vi "Test.vi"() -> ()   [LabVIEW 2017]
uses:
  <instrlib>/Mercury iXX/Public/Controls/Comms Transport Layer.ctl
  <instrlib>/Mercury iXX/Public/Controls/Unit String.ctl
  <instrlib>/Mercury iXX/Public/Libraries/System/Open/Open System.vi
  <instrlib>/Mercury iXX/Public/Libraries/System/Read/Catalogue (Read).vi
  <instrlib>/Mercury iXX/Public/Libraries/Temperature/Open/Open Temperature Device.vi
  <instrlib>/Mercury iXX/Public/Libraries/Temperature/Signals/Read/Temperature (Read).vi
  <vilib>/Utility/file.llb/Write Delimited Spreadsheet (string).vi
  ProgramData/Documents/Princeton Instruments/LightField/Add-in and Automation SDK/Samples/LabVIEW Automation/lightfield-automation-labview/LightField Automation.lvclass
  <instrlib>/Mercury iXX/Mercury iXX.lvlib
  <instrlib>/Quantum Composers 9000 Series 2.08/Quantum Composers 9000 Series.lvlib
  <instrlib>/Mercury iXX/Public/Libraries/Temperature.lvlib
  <instrlib>/Mercury iXX/Public/Libraries/System.lvlib
  <instrlib>/Tektronix TDS 200 1000 2000 Series/Tektronix TDS 200 1000 2000 Series.lvlib
  <instrlib>/Tektronix TDS 200 1000 2000 Series/Public/Data/Read (Multiple Waveforms).vi
  <vilib>/Waveform/WDTFileIO.llb/ Write Waveforms to File (1D).vi
  <vilib>/Waveform/WDTFileIO.llb/Export Waveforms To Spreadsheet File (1D).vi
  <instrlib>/Tektronix TDS 200 1000 2000 Series/Public/Configure/Configure Trigger (Edge).vi
panel:
  out "Array":string[](array[string])
  out "Array 2":string[](array[string])
  in  "?":bool
  in  "Turbulence Experiment":T1(tab)
  in  "VISA resource name":refnum<visa-resource-name>
  in  "Comms Layer":T2
  in  "Device Identifier":string="MB1.T1:TEMP"
  out "error out":errorcluster
  in  "Read Interval (s)":sgl=1.0 min=0.25 max=1000 step=0.25 format="%.2f"
  in  "Record Temperature Data":bool
  out "Unit":T3
  out "Temperature":dbl
  in  "Experiment Name":string="Experiment1"
  in  "Repetitive Gate Width (us)":dbl
  in  "Intensifier Gain":i32
  in  "Start":bool
  in  "?":bool
  in  "Time between frames":i32=500
  in  "On Chip Accumulations 2":i32=6
  in  "Number of Frames 2":i32
  in  "COM Port Settings":T4={"Unit ID"="A", "Baud Rate"=enum."19200", "VISA Sesssion In"="COM1"}
  out "Measurement Data":T5
  in  "Minimum time between \nreadings [ms]":u32
  out "Elapsed Time [ms]":dbl caption="Elapsed Time (s)"
  out "Measurements\nper second":dbl
  in  "End Program":bool
  out "Error Text":string
  out "Error Present":bool
  out "Range Exceeded":bool
  in  "Data Logging Options (If valid)":T6={"Absolute Press."=TRUE, "Gauge/Diff. Press."=TRUE, "Barometric Press."=TRUE, "Temperature"=TRUE, "Volumetric"=TRUE, "Mass Flow"=TRUE, "Setpoint"=TRUE, "Valve Drive"=FALSE, "Totalizer"=TRUE, "Tot. Timer [s]"=FALSE, "Tot. Avg. Flow"=FALSE, "Tot. Peak Flow"=FALSE, "Gas Selected"=TRUE, "Log Data"=TRUE}
  out "Commands":string
  in  "OK Button":bool
  in  "Command to Send":string
  out "Response from Alicat":string
  in  "End Program 2":bool
  in  "Data folder":path=path "C:/Data"
  in  "Oscilloscope":refnum<visa-resource-name>="USB0::0x0699::0x03A6::C016710::INSTR"
  in  "Pulse generater":refnum<visa-resource-name>="COM3"
  # "Stop Oscilloscope"
  # "Stop Lightfield"
  # "Totalizer Timer"
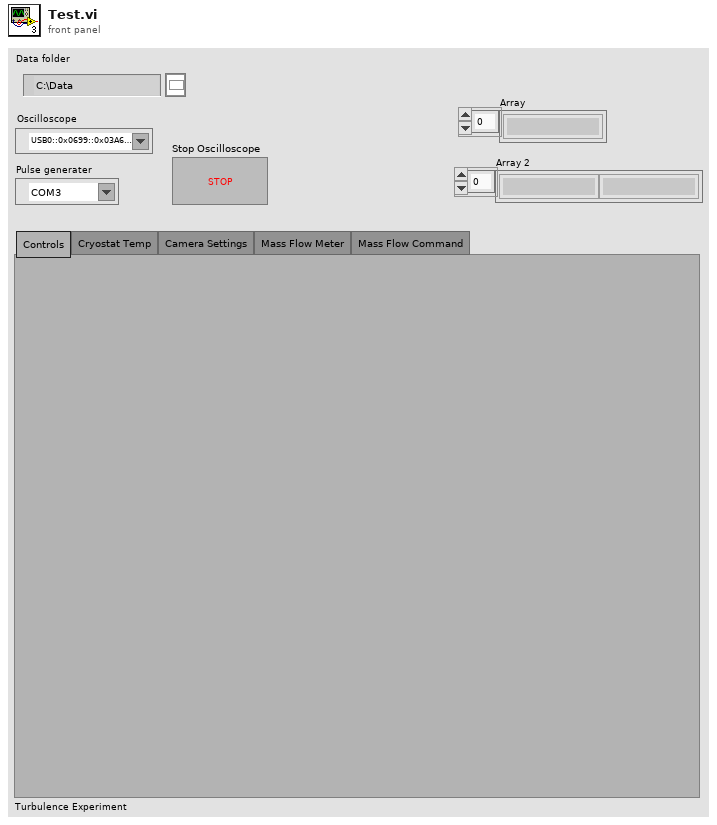
[diagram p1: front panel]
types:
  T1 = enum32{"Controls", "Cryostat Temp", "Camera Settings", "Mass Flow Meter", "Mass Flow Command"}
  T2 = typedef "Mercury iXX.lvlib/Comms Transport Layer.ctl" = enum16{"Ethernet TCP/IP", "USB", "ISOBus - RS-232", "GPIB"}
  T3 = typedef "Mercury iXX.lvlib/Unit String.ctl" = string
  T4 = cluster{"Unit ID":string, "Baud Rate":enum8{"2400", "9600", "19200", "38400", "57600", "115200", "Unknown"}, "VISA Sesssion In":refnum<visa-resource-name>}
  T5 = cluster{"Absolute Pressure":dbl, "Gauge/Diff. Pressure":dbl, "Barometric Pressure":dbl, "Temperature":dbl, "Volumetric Flow":dbl, "Mass Flow":dbl, "Setpoint":dbl, "Valve Drive":dbl, "Totalizer":dbl, "[hr]":dbl, "[min]":dbl, "[sec]":dbl, "Totalizer Average Flow":dbl, "Totalizer Peak Flow":dbl, "Gas selected":string}
  T6 = cluster{"Absolute Press.":bool, "Gauge/Diff. Press.":bool, "Barometric Press.":bool, "Temperature":bool, "Volumetric":bool, "Mass Flow":bool, "Setpoint":bool, "Valve Drive":bool, "Totalizer":bool, "Tot. Timer [s]":bool, "Tot. Avg. Flow":bool, "Tot. Peak Flow":bool, "Gas Selected":bool, "Log Data":bool}
  T7 = typedef "Mercury iXX.lvlib/Mercury Reference.ctl" = cluster{"Comms":refnum<visa-resource-name>, "Device ID":string[], "Comms Layer":T2, "Command":string, "Query reference":T8}
  T8 = typedef "Mercury iXX.lvlib/Query Dynamic Reference.ctl" = refnum<vi>
  T9 = enum16{"open", "replace", "create", "open or create", "replace or create", "replace or create with confirmation"}
  T10 = cluster{"Absolute Pressure":bool, "Gauge/Diff. Pressure":bool, "Barometric Pressure":bool, "Temperature":bool, "Volumetric":bool, "Mass":bool, "Setpoint":bool, "Valve Drive":bool, "Totalizer":bool, "Totalizer Timer":bool, "Totalizer Average Flow":bool, "Totalizer Peak Flow":bool, "Gas Selected":bool, "Tot. Timer Format":u16}
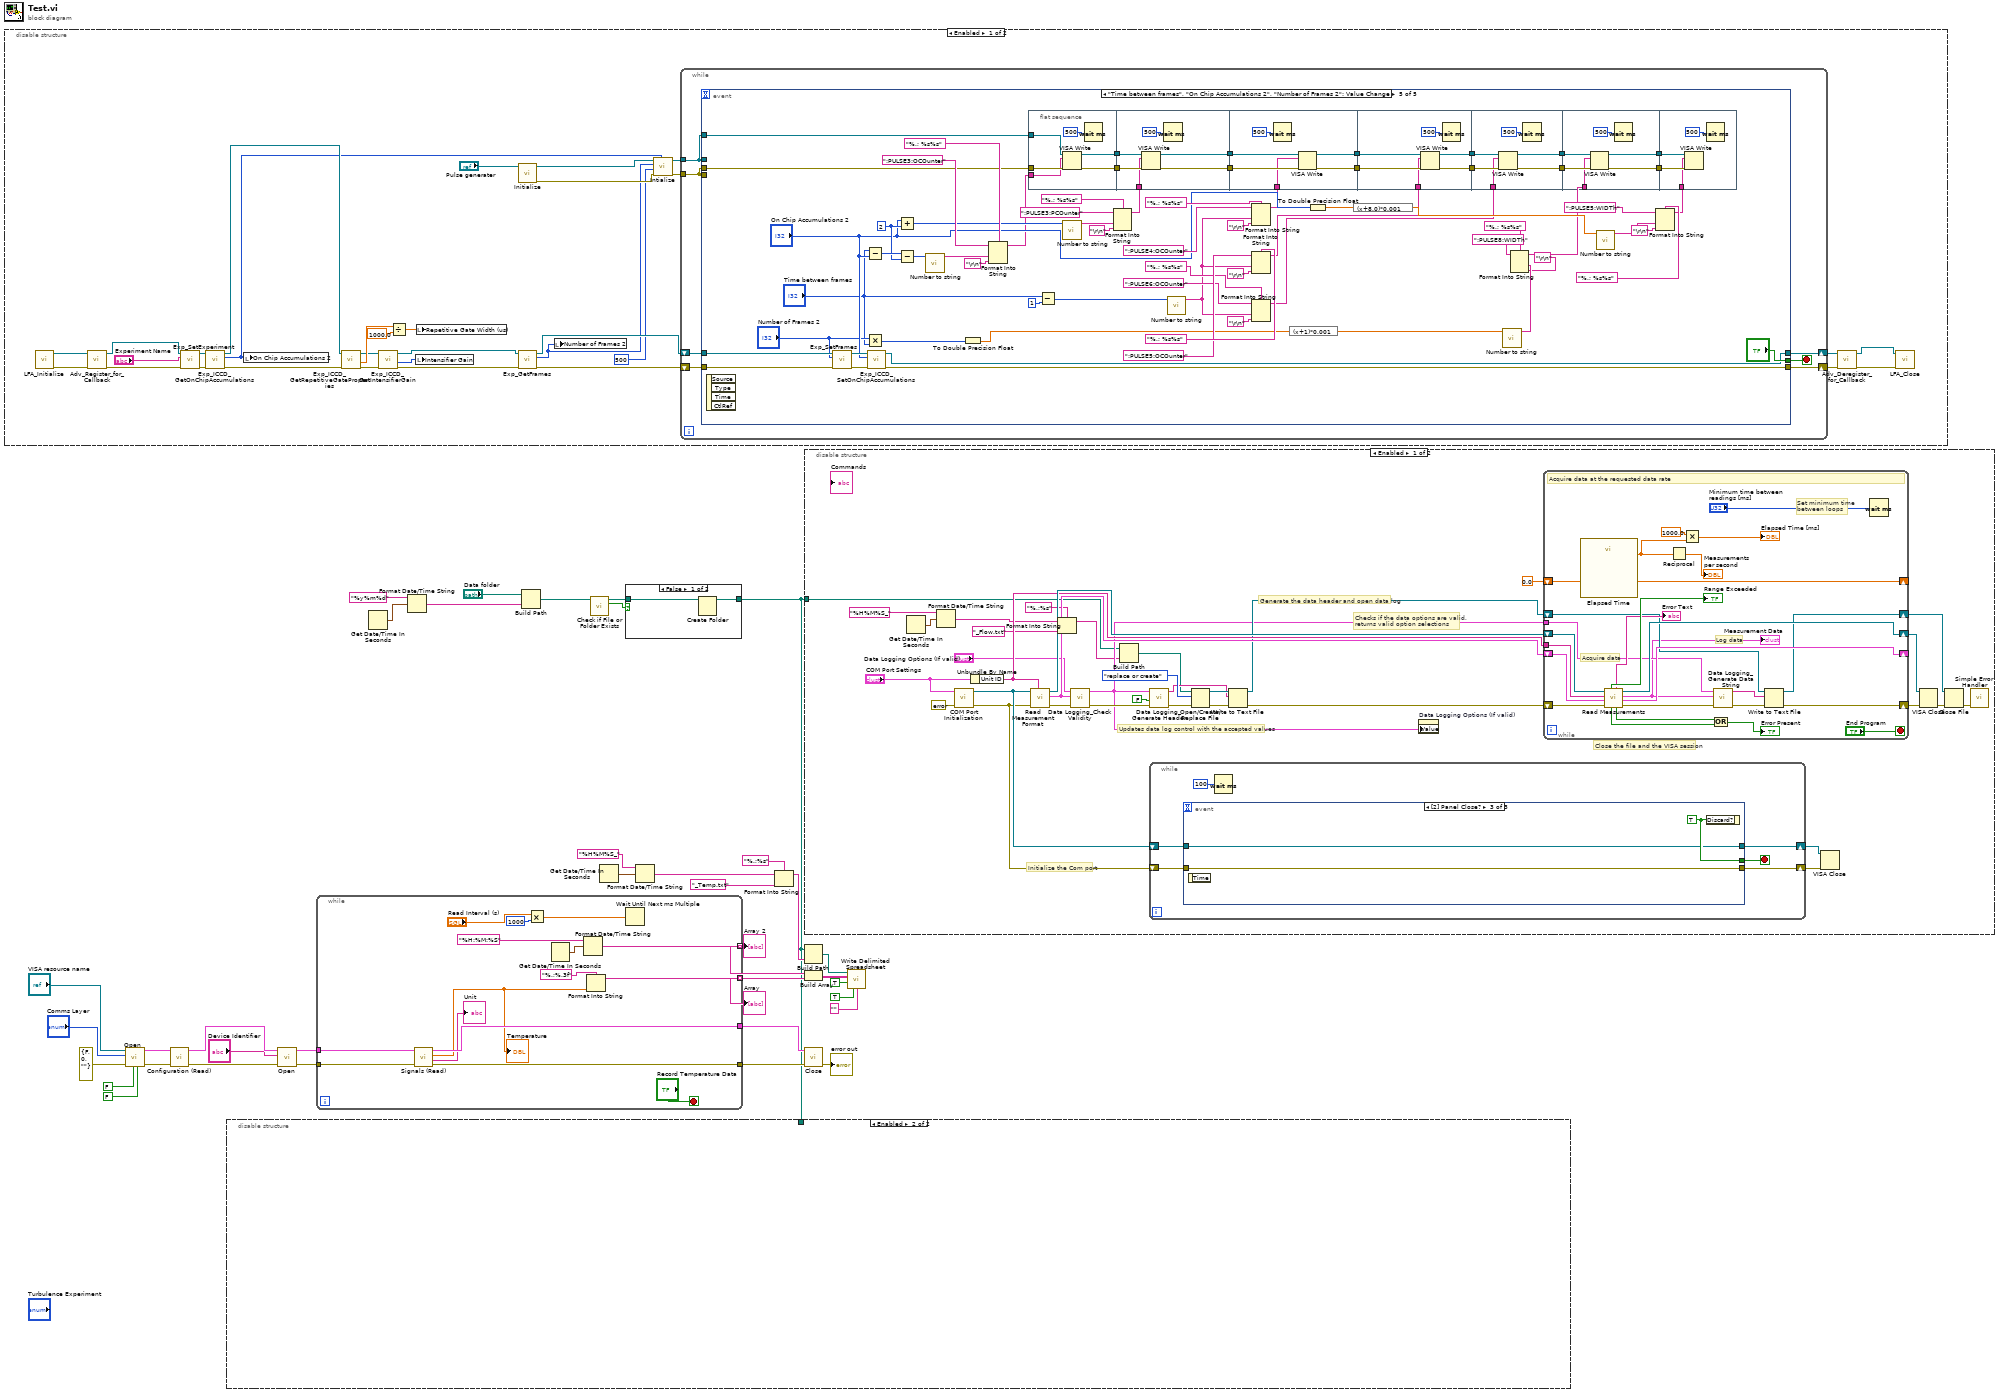
[diagram p0: block diagram]
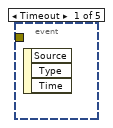
[diagram p2: hidden frame]
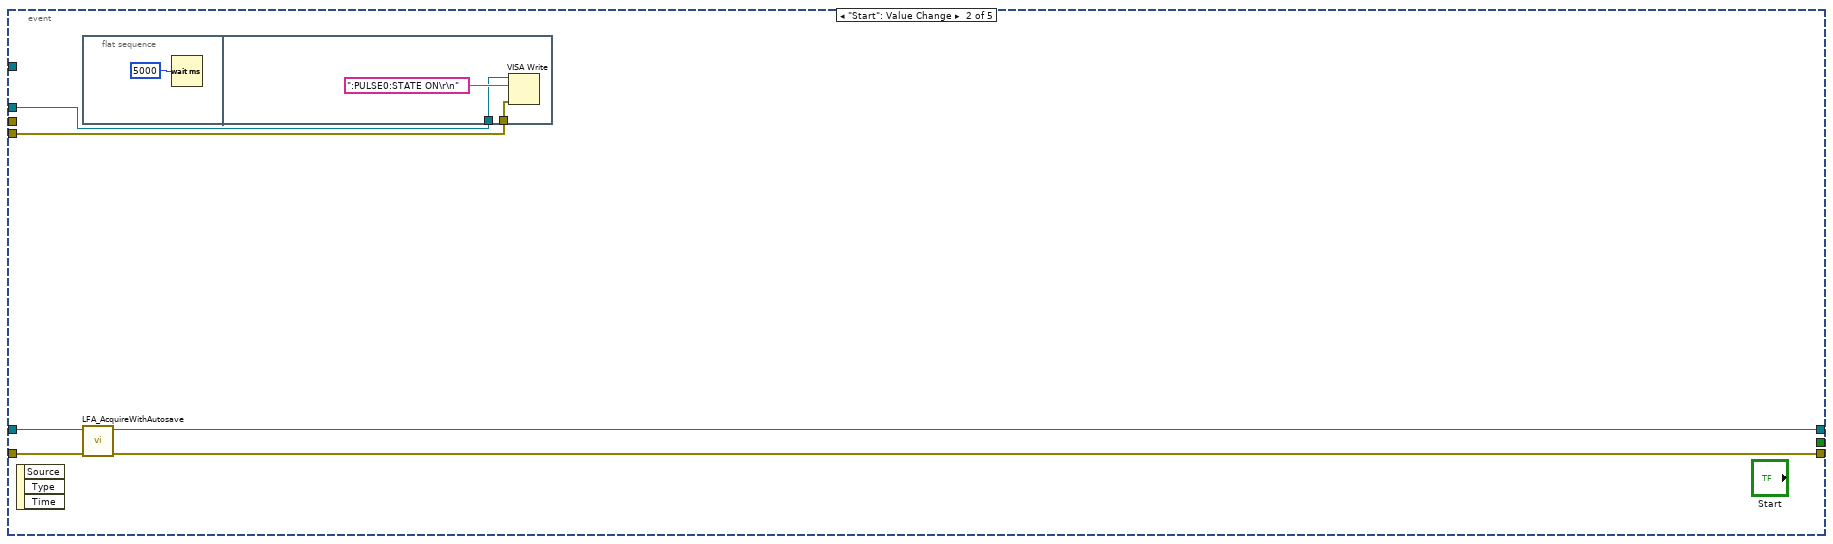
[diagram p3: hidden frame]
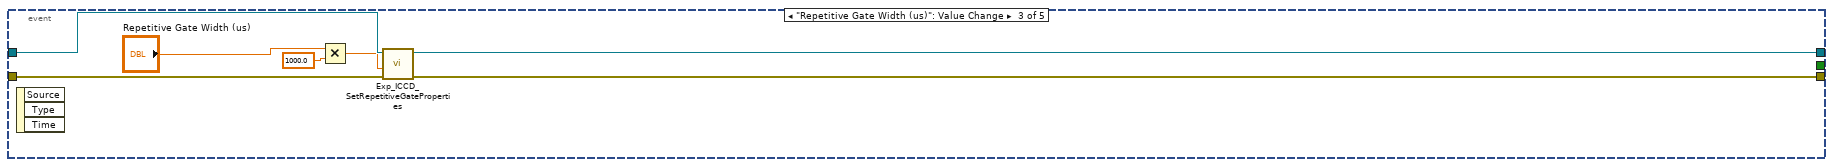
[diagram p4: hidden frame]
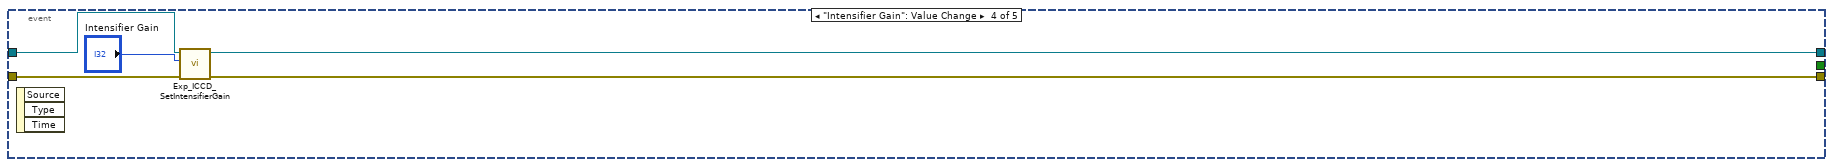
[diagram p5: hidden frame]
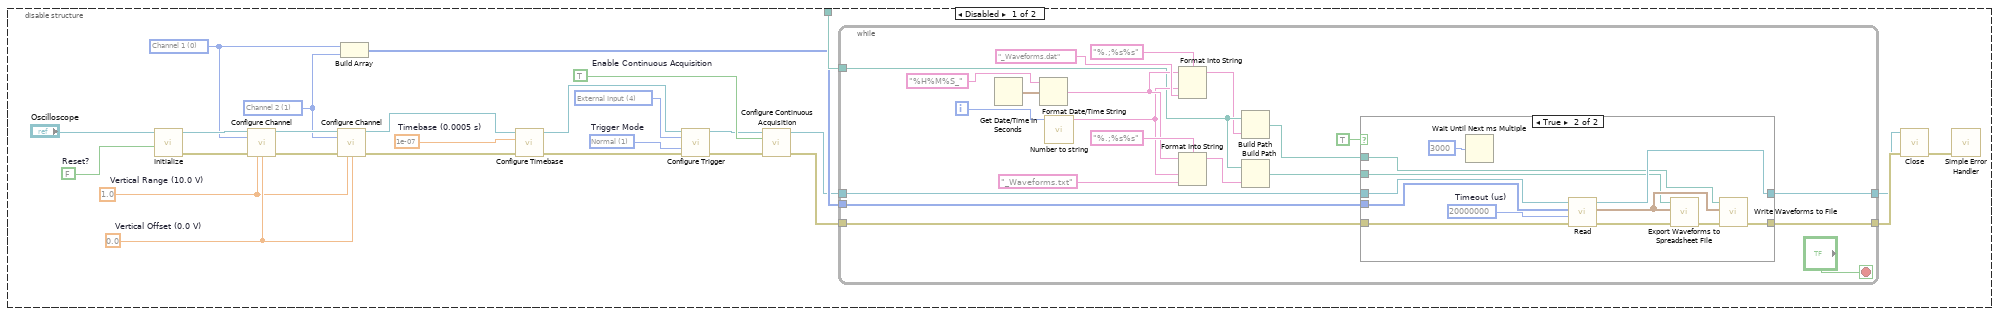
[diagram p7: hidden frame]
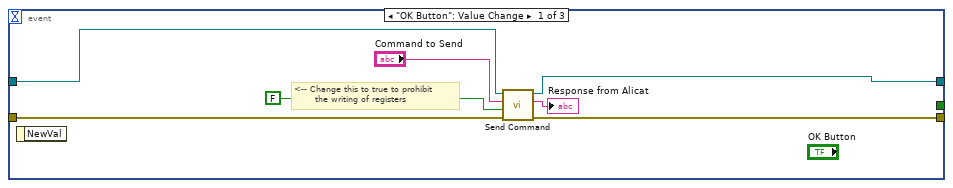
[diagram p9: hidden frame]
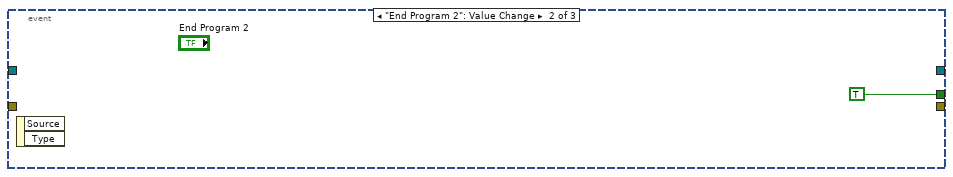
[diagram p10: hidden frame]
diagram:
  n1 = disable-structure shown="Enabled" {
    frame Enabled {
      n2 = call "LFA_Initialize.vi"() -> ("error out"=w37:errorcluster, "LightField Automation out"=w38:refnum<class "LightField Automation.lvclass">)  [unwired: 10 in]
      n3 = call "Adv_Register_for_Callback.vi"("error in (no error)"=w37, "LightField Automation in"=w38) -> ("error out"=w63:errorcluster, "LightField Automation out"=w64:refnum<class "LightField Automation.lvclass">)  [unwired: 8 in]
      n4 = call "Exp_SetExperiment.vi"("error in (no error)"=w63, "ExperimentName"="Experiment Name", "LightField Automation in"=w64) -> ("error out"=w59:errorcluster, "LightField Automation out"=w60:refnum<class "LightField Automation.lvclass">)  [unwired: 7 in]
      n5 = call "Exp_ICCD_GetOnChipAccumulations.vi"("error in (no error)"=w59, "LightField Automation in"=w60) -> ("error out"=w57:errorcluster, "On Chip Accumulations"=w41:i32, "LightField Automation out"=w58:refnum<class "LightField Automation.lvclass">)  [unwired: 7 in]
      n6 = local write "On Chip Accumulations 2"(w41) -> ()
      n7 = call "Exp_ICCD_GetRepetitiveGateProperties.vi"("error in (no error)"=w57, "LightField Automation in"=w58) -> ("error out"=w52:errorcluster, "Repetitive Gate Width (ns)"=w56:dbl, "LightField Automation out"=w53:refnum<class "LightField Automation.lvclass">)  [unwired: 6 in, 1 out]
      n8 = call "Exp_ICCD_GetIntensifierGain.vi"("error in (no error)"=w52, "LightField Automation in"=w53) -> ("error out"=w49:errorcluster, "Intensifier Gain"=w51:i32, "LightField Automation out"=w50:refnum<class "LightField Automation.lvclass">)  [unwired: 7 in]
      n9 = Divide(x=w56, y=1000.0) -> (x/y=w54:dbl)
      n10 = local write "Intensifier Gain"(w51) -> ()
      n11 = local write "Repetitive Gate Width (us)"(w54) -> ()
      n12 = call <instrlib>:"Initialize.vi"("VISA resource name"="Pulse generater") -> ("error out"=w45:errorcluster, "VISA resource name out"=w46:refnum<visa-resource-name>)  [unwired: 9 in]
      n13 = call "Exp_GetFrames.vi"("error in (no error)"=w49, "LightField Automation in"=w50) -> ("error out"=w48:errorcluster, "Frames"=w42:i32, "LightField Automation out"=w47:refnum<class "LightField Automation.lvclass">)  [unwired: 7 in]
      n14 = local write "Number of Frames 2"(w42) -> ()
      n15 = call "Intialize.vi"("On Chip Accumulations 3"=w41, "error in (no error)"=w45, "Time between frames 2"=500, "Number of Frames 3"=w42, "VISA resource name"=w46) -> ("error out"=w43:errorcluster, "VISA resource name out"=w44:refnum<visa-resource-name>)  [unwired: 5 in]
      n16 = while {
        tunnel: w44 -> [w68]
        tunnel: w43 -> [w69]
        shift-right: [w73] -> w62
        shift-left: w47 -> [w71]
        shift-right: [w74] -> w61
        shift-left: w48 -> [w72]
        stop <- w70 stop-if-true
        n17 = event shown="[4] \"Time between frames\", \"On Chip Accumulations 2\", \"Number of Frames 2\": Value Change" {
          selector: _ -> [_ _ _ _ _]
          dyn-events: _ -> [_ _ _ _ _]
          timeout: _ -> [_ _ _ _ _]
          tunnel: w69 -> [_ w80 _ _ _]
          tunnel: w68 -> [_ w77 _ _ _]
          tunnel: w72 -> [_ w79 w90 w94 w132]
          tunnel: w71 -> [_ w78 w91 w95 w133]
          tunnel: [_ w75 w88 w92 w128] -> w74
          tunnel: [_ w76 w89 w93 w129] -> w73
          tunnel: [_ _ _ _ "?"] -> w70
          tunnel: w69 -> [_ _ _ _ w117]
          tunnel: w68 -> [_ _ _ _ w115]
          event Timeout {
            n18 = event-data() -> ()  [unwired: 1 in, 3 out]
          }
          event "Start": Value Change {
            n19 = event-data() -> ()  [unwired: 1 in, 3 out]
            n20 = flat-sequence {
              tunnel: w80 -> [w84]
              tunnel: w77 -> [w82]
              frame #0 {
                n21 = Wait (ms)(milliseconds to wait=5000) -> ()  [unwired: 1 out]
              }
              frame #1 {
                n22 = VISA Write(VISA resource name=w82, write buffer=":PULSE0:STATE ON\r\n" ("format string"), error in (no error)=w84) -> ()  [unwired: 3 out]
              }
            }
            n23 = call "LFA_AcquireWithAutosave.vi"("error in (no error)"=w79, "LightField Automation in"=w78) -> ("error out"=w75:errorcluster, "LightField Automation out"=w76:refnum<class "LightField Automation.lvclass">)  [unwired: 7 in, 1 out]
          }
          event "Repetitive Gate Width (us)": Value Change {
            n24 = event-data() -> ()  [unwired: 1 in, 3 out]
            n25 = Multiply(x="Repetitive Gate Width (us)", y=1000.0) -> (x*y=w85:dbl)
            n26 = call "Exp_ICCD_SetRepetitiveGateProperties.vi"("error in (no error)"=w90, "Repetitive Gate Width (ns)"=w85, "LightField Automation in"=w91) -> ("error out"=w88:errorcluster, "LightField Automation out"=w89:refnum<class "LightField Automation.lvclass">)  [unwired: 7 in]
          }
          event "Intensifier Gain": Value Change {
            n27 = event-data() -> ()  [unwired: 1 in, 3 out]
            n28 = call "Exp_ICCD_SetIntensifierGain.vi"("error in (no error)"=w94, "Intensifier Gain"="Intensifier Gain", "LightField Automation in"=w95) -> ("error out"=w92:errorcluster, "LightField Automation out"=w93:refnum<class "LightField Automation.lvclass">)  [unwired: 7 in]
          }
          event "Time between frames", "On Chip Accumulations 2", "Number of Frames 2": Value Change {
            w157 = 2 ("y")
            n29 = event-data() -> ()  [unwired: 1 in, 4 out]
            n30 = call "Exp_SetFrames.vi"("error in (no error)"=w132, "Number of Frames"="Number of Frames 2", "LightField Automation in"=w133) -> ("error out"=w130:errorcluster, "LightField Automation out"=w131:refnum<class "LightField Automation.lvclass">)  [unwired: 7 in]
            n31 = Subtract(x="Time between frames", y="On Chip Accumulations 2") -> (x-y=w159:i32)
            n32 = Multiply(x="Number of Frames 2", y="Time between frames") -> (x*y=w118:i32)
            n33 = call "Exp_ICCD_SetOnChipAccumulations.vi"("error in (no error)"=w130, "On Chip Accumulations"="On Chip Accumulations 2", "LightField Automation in"=w131) -> ("error out"=w128:errorcluster, "LightField Automation out"=w129:refnum<class "LightField Automation.lvclass">)  [unwired: 7 in]
            n34 = Add(x="On Chip Accumulations 2", y=w157) -> (x+y=w153:i32)
            n35 = Subtract(x=w159, y=w157) -> (x-y=w158:i32)
            n36 = call "Number to string.vi"("Numeric"=w158) -> ("Shortest String"=w163:string)  [unwired: 10 in]
            n37 = To Double Precision Float(number=w118) -> (double precision float=w139:dbl)
            n38 = Format Into String(format string="%.; %s%s", initial string=":PULSE3:OCOunter" ("format string"), w163, "\r\n" ("format string")) -> (resulting string=w116:string)  [unwired: 1 in, 1 out]
            n39 = flat-sequence {
              tunnel: w117 -> [w170]
              tunnel: w116 -> [w169]
              tunnel: w115 -> [w168]
              tunnel: [w167] -> w114
              tunnel: [w166] -> w112
              tunnel: w114 -> [w175]
              tunnel: w113 -> [w174]
              tunnel: w112 -> [w173]
              tunnel: [w172] -> w111
              tunnel: [w171] -> w109
              tunnel: w111 -> [w182]
              tunnel: w110 -> [w181]
              tunnel: w109 -> [w180]
              tunnel: [w179] -> w108
              tunnel: [w178] -> w106
              tunnel: w108 -> [w188]
              tunnel: w107 -> [w187]
              tunnel: w106 -> [w186]
              tunnel: [w185] -> w105
              tunnel: [w184] -> w103
              tunnel: w105 -> [w194]
              tunnel: w104 -> [w193]
              tunnel: w103 -> [w192]
              tunnel: [w191] -> w102
              tunnel: [w190] -> w100
              tunnel: w102 -> [w200]
              tunnel: w101 -> [w199]
              tunnel: w100 -> [w198]
              tunnel: [w197] -> w99
              tunnel: [w196] -> w97
              tunnel: w99 -> [w204]
              tunnel: w98 -> [w203]
              tunnel: w97 -> [w202]
              frame #0 {
                n40 = VISA Write(VISA resource name=w168, write buffer=w169, error in (no error)=w170) -> (VISA resource name out=w166:refnum<visa-resource-name>, error out=w167:errorcluster)  [unwired: 1 out]
                n41 = Wait (ms)(milliseconds to wait=500) -> ()  [unwired: 1 out]
              }
              frame #1 {
                n42 = VISA Write(VISA resource name=w173, write buffer=w174, error in (no error)=w175) -> (VISA resource name out=w171:refnum<visa-resource-name>, error out=w172:errorcluster)  [unwired: 1 out]
                n43 = Wait (ms)(milliseconds to wait=500) -> ()  [unwired: 1 out]
              }
              frame #2 {
                n44 = Wait (ms)(milliseconds to wait=500) -> ()  [unwired: 1 out]
                n45 = VISA Write(VISA resource name=w180, write buffer=w181, error in (no error)=w182) -> (VISA resource name out=w178:refnum<visa-resource-name>, error out=w179:errorcluster)  [unwired: 1 out]
              }
              frame #3 {
                n46 = VISA Write(VISA resource name=w186, write buffer=w187, error in (no error)=w188) -> (VISA resource name out=w184:refnum<visa-resource-name>, error out=w185:errorcluster)  [unwired: 1 out]
                n47 = Wait (ms)(milliseconds to wait=500) -> ()  [unwired: 1 out]
              }
              frame #4 {
                n48 = VISA Write(VISA resource name=w192, write buffer=w193, error in (no error)=w194) -> (VISA resource name out=w190:refnum<visa-resource-name>, error out=w191:errorcluster)  [unwired: 1 out]
                n49 = Wait (ms)(milliseconds to wait=500) -> ()  [unwired: 1 out]
              }
              frame #5 {
                n50 = VISA Write(VISA resource name=w198, write buffer=w199, error in (no error)=w200) -> (VISA resource name out=w196:refnum<visa-resource-name>, error out=w197:errorcluster)  [unwired: 1 out]
                n51 = Wait (ms)(milliseconds to wait=500) -> ()  [unwired: 1 out]
              }
              frame #6 {
                n52 = VISA Write(VISA resource name=w202, write buffer=w203, error in (no error)=w204) -> ()  [unwired: 3 out]
                n53 = Wait (ms)(milliseconds to wait=500) -> ()  [unwired: 1 out]
              }
            }
            n54 = Subtract(x="Time between frames", y=1) -> (x-y=w150:i32)
            n55 = call "Number to string.vi"("Numeric"=w153) -> ("Shortest String"=w156:string)  [unwired: 10 in]
            n56 = Format Into String(format string="%.; %s%s", initial string=":PULSE3:PCOunter" ("format string"), w156, "\r\n" ("format string")) -> (resulting string=w113:string)  [unwired: 1 in, 1 out]
            n57 = call "Number to string.vi"("Numeric"=w150) -> ("Shortest String"=w140:string)  [unwired: 10 in]
            n58 = Format Into String(format string="%.; %s%s", initial string=":PULSE4:OCOunter" ("format string"), w140, "\r\n" ("format string")) -> (resulting string=w110:string)  [unwired: 1 in, 1 out]
            n59 = Format Into String(format string="%.; %s%s", initial string=":PULSE5:OCOunter" ("format string"), w140, "\r\n" ("format string")) -> (resulting string=w107:string)  [unwired: 1 in, 1 out]
            n60 = Format Into String(format string="%.; %s%s", initial string=":PULSE6:OCOunter" ("format string"), w140, "\r\n" ("format string")) -> (resulting string=w104:string)  [unwired: 1 in, 1 out]
            n61 = expression code="(x+1)*0.001"(w139) -> (w136:dbl)
            n62 = To Double Precision Float(number="On Chip Accumulations 2") -> (double precision float=w126:dbl)
            n63 = expression code="(x+8.0)*0.001"(w126) -> (w121:dbl)
            n64 = call "Number to string.vi"("Numeric"=w136) -> ("Shortest String"=w135:string)  [unwired: 10 in]
            n65 = Format Into String(format string="%.; %s%s", initial string=":PULSE8:WIDTh" ("format string"), w135, "\r\n" ("format string")) -> (resulting string=w101:string)  [unwired: 1 in, 1 out]
            n66 = call "Number to string.vi"("Numeric"=w121) -> ("Shortest String"=w123:string)  [unwired: 10 in]
            n67 = Format Into String(format string="%.; %s%s", initial string=":PULSE5:WIDTh" ("format string"), w123, "\r\n" ("format string")) -> (resulting string=w98:string)  [unwired: 1 in, 1 out]
          }
        }
      }
      n68 = call "Adv_Deregister_for_Callback.vi"("error in (no error)"=w61, "LightField Automation in"=w62) -> ("error out"=w39:errorcluster, "LightField Automation out"=w66:refnum<class "LightField Automation.lvclass">)  [unwired: 8 in]
      n69 = call "LFA_Close.vi"("error in (no error)"=w39, "LightField Automation in"=w66) -> ()  [unwired: 8 in, 2 out]
    }
    frame Disabled {
    }
  }
  n70 = call-poly <instrlib>:"Open.vi"("Clear Previous Connections (False)"=FALSE, "ID Query (True)"=FALSE, "error in (no error)"=errorcluster {"status"=FALSE, "code"=0, "source"=""}, "Comms Layer"="Comms Layer", "VISA resource name"="VISA resource name") -> ("error out"=w26:errorcluster, "Mercury Reference Out"=w27:T7)  [unwired: 2 in, 3 out]
  n71 = call-poly <instrlib>:"Configuration (Read).vi"("error in"=w26, "Mercury Reference In"=w27) -> ("error out"=w24:errorcluster, "Mercury Reference Out"=w25:T7)  [unwired: 6 in, 2 out]
  n72 = call-poly <instrlib>:"Open.vi"("error in (no error)"=w24, "Device Identifier"="Device Identifier", "Mercury Reference In"=w25) -> ("error out"=w21:errorcluster, "Mercury Reference Out"=w22:T7)  [unwired: 7 in]
  n73 = while {
    tunnel: w22 -> [w219]
    tunnel: w21 -> [w218]
    tunnel: [w217] -> w20
    tunnel: [w216] -> w19
    tunnel: [w205] -> w13 mode=indexing
    tunnel: [w208] -> w14 mode=indexing
    stop <- "Record Temperature Data" stop-if-true
    n74 = call-poly <instrlib>:"Signals (Read).vi"("error in"=w218, "Mercury Reference In"=w219) -> ("error out"=w217:errorcluster, "Unit"=→"Unit":T3, "Temperature"=w206:dbl, "Mercury Reference Out"=w216:T7)  [unwired: 5 in, 1 out]
    "Temperature" <- w206
    n75 = Multiply(x="Read Interval (s)", y=u32 1000 ("millisecond multiple")) -> (x*y=w211:sgl)
    n76 = Get Date/Time In Seconds() -> (seconds since 1Jan1904=w209:timestamp)
    n77 = Format Date/Time String(time format string (%c)="%H:%M:%S", seconds (now)=w209) -> (date/time string=w208:string)  [unwired: 1 in]
    n78 = Format Into String(format string="%.;%.3f", w206) -> (resulting string=w205:string)  [unwired: 2 in, 1 out]
    n79 = Wait Until Next ms Multiple(millisecond multiple=w211) -> ()  [unwired: 1 out]
  }
  "Array 2" <- w14
  "Array" <- w13
  n80 = Get Date/Time In Seconds() -> (seconds since 1Jan1904=w34:timestamp)
  n81 = Format Date/Time String(time format string (%c)="%y%m%d", seconds (now)=w34) -> (date/time string=w33:string)  [unwired: 1 in]
  n82 = Build Path(base path="Data folder", name or relative path=w33) -> (appended path=w32:path)
  n83 = call <vilib>:"Check if File or Folder Exists.vi"("path"=w32) -> ("file or folder exists?"=w30:bool, "dup path"=w31:path)  [unwired: 8 in, 1 out]
  n84 = Get Date/Time In Seconds() -> (seconds since 1Jan1904=w11:timestamp)
  n85 = case shown="False" w30 {
    tunnel: w31 -> [w221 w222]
    tunnel: [w220 w222] -> w1
    frame False {
      n86 = Create Folder(path (use dialog)=w221) -> (created path=w220:path)  [unwired: 2 in, 2 out]
    }
    frame True {
    }
  }
  n87 = disable-structure shown="Enabled" {
    disable-tunnel: w1 -> [w249 _]
    frame Disabled {
      w226 = 1 items=["Channel 1", "Channel 2", "Channel 3", "Channel 4", "Math", "Reference A", "Reference B", "Reference C", "Reference D"] ("Channel (0: Channel 1)")
      w225 = 0 items=["Channel 1", "Channel 2", "Channel 3", "Channel 4", "Math", "Reference A", "Reference B", "Reference C", "Reference D"] ("Channel (0: Channel 1)")
      w233 = 4 items=["Channel 1", "Channel 2", "Channel 3", "Channel 4", "External Input", "Attenuated External Input"] ("Trigger Source (0: Channel 1)")
      w242 = u16 1 items=["Auto", "Normal"]  # Trigger Mode
      w243 = FALSE  # Reset?
      w224 = 0.0  # Vertical Offset (0.0 V)
      w248 = 1e-07  # Timebase (0.0005 s)
      w223 = 1.0  # Vertical Range (10.0 V)
      w244 = TRUE  # Enable Continuous Acquisition
      n88 = call <instrlib>:"Initialize.vi"("Reset? (T: Yes)"=w243, "VISA resource name"="Oscilloscope") -> ("error out"=w245:errorcluster, "VISA resource name out"=w246:refnum<visa-resource-name>)  [unwired: 3 in, 5 out]
      n89 = call <instrlib>:"Configure Channel.vi"("VISA resource name"=w246, "Channel (0: Channel 1)"=w225, "error in (no error)"=w245, "Vertical Range (10.0 V/div)"=w223, "Vertical Offset (0.0 divs)"=w224) -> ("VISA resource name out"=w237:refnum<visa-resource-name>, "error out"=w236:errorcluster)  [unwired: 4 in, 5 out]
      n90 = call <instrlib>:"Configure Channel.vi"("VISA resource name"=w237, "Channel (0: Channel 1)"=w226, "error in (no error)"=w236, "Vertical Range (10.0 V/div)"=w223, "Vertical Offset (0.0 divs)"=w224) -> ("VISA resource name out"=w235:refnum<visa-resource-name>, "error out"=w234:errorcluster)  [unwired: 4 in, 5 out]
      n91 = Build Array(w225, w226) -> (w230:i32[])
      n92 = call <instrlib>:"Configure Timebase.vi"("error in (no error)"=w234, "Timebase (0.0005 s)"=w248, "VISA resource name"=w235) -> ("error out"=w240:errorcluster, "VISA resource name out"=w241:refnum<visa-resource-name>)  [unwired: 1 in, 6 out]
      n93 = call-poly <instrlib>:"Configure Trigger.vi"("VISA resource name"=w241, "Trigger Source (0: Channel 1)"=w233, "Trigger Mode (0: Auto)"=w242, "error in (no error)"=w240) -> ("VISA resource name out"=w239:refnum<visa-resource-name>, "error out"=w238:errorcluster)  [unwired: 4 in, 6 out]
      n94 = call <instrlib>:"Configure Continuous Acquisition.vi"("error in (no error)"=w238, "Enable Continuous Acquisition Mode (True)"=w244, "VISA resource name"=w239) -> ("error out"=w231:errorcluster, "VISA resource name out"=w229:refnum<visa-resource-name>)  [unwired: 7 out]
      n95 = while {
        tunnel: w231 -> [w270]
        tunnel: w230 -> [w269]
        tunnel: w229 -> [w268]
        tunnel: [w267] -> w228
        tunnel: [w266] -> w227
        tunnel: w249 -> [w253]
        i -> [w259]
        stop <- "?" stop-if-true
        n96 = Get Date/Time In Seconds() -> (seconds since 1Jan1904=w263:timestamp)
        n97 = Format Date/Time String(time format string (%c)="%H%M%S_", seconds (now)=w263) -> (date/time string=w256:string)  [unwired: 1 in]
        n98 = call "Number to string.vi"("Numeric"=w259) -> ("Shortest String"=w255:string)  [unwired: 10 in]
        n99 = Format Into String(format string="%.;%s%s", initial string=w256, w255, "_Waveforms.dat" ("input 2")) -> (resulting string=w252:string)  [unwired: 1 in, 1 out]
        n100 = Format Into String(format string="%.;%s%s", initial string=w256, w255, "_Waveforms.txt" ("input 2")) -> (resulting string=w261:string)  [unwired: 1 in, 1 out]
        n101 = Build Path(base path=w253, name or relative path=w252) -> (appended path=w251:path)
        n102 = Build Path(base path=w253, name or relative path=w261) -> (appended path=w254:path)
        n103 = case shown="True" TRUE {
          tunnel: w270 -> [w271 w284]
          tunnel: w269 -> [_ w283]
          tunnel: w268 -> [w272 w282]
          tunnel: [w271 w276] -> w267
          tunnel: [w272 w281] -> w266
          tunnel: w254 -> [_ w275]
          tunnel: w251 -> [_ w274]
          frame False {
          }
          frame True {
            w273 = u32 20000000  # Timeout (us)
            n104 = Wait Until Next ms Multiple(millisecond multiple=u32 3000) -> ()  [unwired: 1 out]
            n105 = call-poly <instrlib>:"Read.vi"("error in (no error)"=w284, "Timeout (10000 ms)"=w273, "Channels"=w283, "VISA resource name"=w282) -> ("error out"=w277:errorcluster, "Waveform Data"=w278:waveform(dbl)[], "VISA resource name out"=w281:refnum<visa-resource-name>)  [unwired: 5 out]
            n106 = call-poly <vilib>:"Export Waveforms to Spreadsheet File.vi"("error in (no error)"=w277, "waveforms"=w278, "file path (dialog if empty)"=w275) -> ("error out"=w279:errorcluster)  [unwired: 7 in, 1 out]
            n107 = call-poly <vilib>:"Write Waveforms to File.vi"("error in (no error)"=w279, "waveform array"=w278, "file path (dialog if empty)"=w274) -> ("error out"=w276:errorcluster)  [unwired: 7 in, 1 out]
          }
        }
      }
      n108 = call <instrlib>:"Close.vi"("error in (no error)"=w228, "VISA resource name"=w227) -> ("error out"=w232:errorcluster)  [unwired: 9 out]
      n109 = call <vilib>:"Simple Error Handler.vi"("error in (no error)"=w232) -> ()  [unwired: 1 in, 8 out]
    }
    frame Enabled {
    }
  }
  n110 = Format Date/Time String(time format string (%c)="%H%M%S_", seconds (now)=w11) -> (date/time string=w7:string)  [unwired: 1 in]
  n111 = Format Into String(format string="%.;%s", initial string=w7, "_Temp.txt" ("input 2")) -> (resulting string=w8:string)  [unwired: 1 in, 1 out]
  n112 = disable-structure shown="Enabled" {
    disable-tunnel: w1 -> [w290 _]
    frame Enabled {
      # "Updates data log control with the accepted values"
      # "Checks if the data options are valid,\nreturns valid option selections"
      # "Generate the data header and open data log"
      # "Close the file and the VISA session"
      # "Initialize the Com port"
      n113 = Get Date/Time In Seconds() -> (seconds since 1Jan1904=w295:timestamp)
      n114 = Format Date/Time String(time format string (%c)="%H%M%S_", seconds (now)=w295) -> (date/time string=w291:string)  [unwired: 1 in]
      n115 = call "COM Port Initialization.vi"("error in (no error)"=errorcluster {"status"=FALSE, "code"=0, "source"=""}, "Communication Settings"="COM Port Settings") -> ("error out"=w285:errorcluster, "VISA Session Out"=w286:refnum<visa-resource-name>)  [unwired: 8 in]
      n116 = Unbundle By Name("COM Port Settings") -> ("Unit ID"=w314:string)
      n117 = call "Read Measurement Format.vi"("Unit ID (A)"=w314, "error in"=w285, "VISA Session In"=w286) -> ("error out"=w305:errorcluster, "Data Frame Format"=w313:T10, "VISA Session Out"=w315:refnum<visa-resource-name>)  [unwired: 6 in]
      n118 = Format Into String(format string="%.;%s", initial string=w291, "_Flow.txt" ("input 2")) -> (resulting string=w292:string)  [unwired: 1 in, 1 out]
      n119 = call "Data Logging_Check Validity.vi"("error in"=w305, "Data Frame Format"=w313, "Data Logging Options (If valid)"="Data Logging Options (If valid)") -> ("error out"=w311:errorcluster, "Validated Logging Options"=w298:T6)  [unwired: 6 in, 1 out]
      n120 = Build Path(base path=w290, name or relative path=w292) -> (appended path=w289:path)
      n121 = while {
        shift-right: [w323] -> w288
        shift-left: w286 -> [w325]
        shift-right: [w322] -> w287
        shift-left: w285 -> [w324]
        stop <- w321 stop-if-true
        n122 = event shown="[2] Panel Close?" {
          selector: _ -> [_ _ _]
          dyn-events: _ -> [_ _ _]
          timeout: _ -> [_ _ _]
          tunnel: w325 -> [w328 _ w334]
          tunnel: w324 -> [w332 _ w335]
          tunnel: [w327 _ w334] -> w323
          tunnel: [w331 _ w335] -> w322
          tunnel: [_ TRUE ("Discard?") w336] -> w321
          event "OK Button": Value Change {
            # "<-- Change this to true to prohibit\n       the writing of registers"
            n123 = event-data() -> ()  [unwired: 1 in, 1 out]
            n124 = call "Send Command.vi"("error in"=w332, "Disable register writing (T)"=FALSE ("Disable register writing"), "Command"="Command to Send", "VISA Session In"=w328) -> ("error out"=w331:errorcluster, "Response"=→"Response from Alicat":string, "VISA Session Out"=w327:refnum<visa-resource-name>)  [unwired: 5 in]
          }
          event "End Program 2": Value Change {
            n125 = event-data() -> ()  [unwired: 1 in, 2 out]
          }
          event Panel Close? {
            w336 = TRUE ("Discard?")
            n126 = event-data() -> ()  [unwired: 1 in, 1 out]
            n127 = event-data("Discard?"=w336) -> ()  [unwired: 1 in, 1 out]
          }
        }
        n128 = Wait (ms)(milliseconds to wait=u32 100) -> ()  [unwired: 1 out]
      }
      n129 = call "Data Logging_Generate Header.vi"("error in"=w311, "Include Units\nin Header (F)"=FALSE ("Include Units\nin Header (default is F)"), "Data Logging Options"=w298) -> ("error out"=w307:errorcluster, "Data Log Header"=w304:string)  [unwired: 7 in]
      n130 = Open/Create/Replace File(file path (use dialog)=w289, error in=w307, operation (0:open)=T9."replace or create") -> (refnum out=w310:refnum<file>, error out=w309:errorcluster)  [unwired: 3 in, 1 out]
      n131 = Write to Text File(file (use dialog)=w310, text=w304, error in=w309) -> (refnum out=w303:refnum<file>, error out=w306:errorcluster)  [unwired: 1 in, 1 out]
      n132 = property on="Data Logging Options (If valid)" class="Clust (strict)"("Value"=w298) -> ()  [unwired: 2 in, 2 out]
      n133 = while {
        shift-right: [w360] -> _
        shift-left: 0.0 ("Set Start Time (s)") -> [w363]
        shift-right: [w340] -> w302
        shift-left: w306 -> [w362]
        shift-right: [w359] -> w316
        shift-left: w315 -> [w361]
        tunnel: w314 -> [w358]
        shift-right: [w352] -> _
        shift-left: w313 -> [w357]
        shift-right: [w338] -> w299
        shift-left: w303 -> [w339]
        tunnel: w298 -> [w344]
        stop <- "End Program" stop-if-true
        # "Log data"
        # "Set minimum time\nbetween loops"
        # "Acquire data"
        # "Acquire data at the requested data rate"
        n134 = call "Elapsed Time"("Set Start Time (s)"=w363) -> ("Get Start Time (s)"=w360:dbl, "Elapsed Time (s)"=w346:dbl)  [unwired: 11 in, 6 out]
        n135 = call "Read Measurements.vi"("error in"=w362, "Data Frame Format In"=w357, "Unit ID (A)"=w358, "VISA Session In"=w361) -> ("error out"=w343:errorcluster, "Data Frame Format Out"=w352:T10, "Data Cluster"=w337:T5, "VISA Session Out"=w359:refnum<visa-resource-name>, "Unknown Dataframe Info"=w356:bool, "Error/Overrange/Unknown String"=→"Error Text":string, "Error Present"=w355:bool, "Range Exceeded"=→"Range Exceeded":bool)
        "Measurement Data" <- w337
        n136 = Reciprocal(x=w346) -> (1/x=→"Measurements\nper second":dbl)
        n137 = Multiply(x=1000.0 ("y"), y=w346) -> (x*y=→"Elapsed Time [ms]":dbl)
        n138 = Or(x=w356, y=w355) -> (x .or. y?=→"Error Present":bool)
        n139 = call "Data Logging_Generate Data String.vi"("error in"=w343, "Measurement Data"=w337, "Data Logging Options"=w344) -> ("error out"=w342:errorcluster, "Data Log String"=w341:string)  [unwired: 6 in, 1 out]
        n140 = Write to Text File(file (use dialog)=w339, text=w341, error in=w342) -> (refnum out=w338:refnum<file>, error out=w340:errorcluster)  [unwired: 1 in, 1 out]
        n141 = Wait (ms)(milliseconds to wait="Minimum time between \nreadings [ms]") -> ()  [unwired: 1 out]
      }
      n142 = VISA Close(VISA resource name=w288, error in (no error)=w287) -> ()  [unwired: 1 out]
      n143 = VISA Close(VISA resource name=w316, error in (no error)=w302) -> (error out=w301:errorcluster)
      n144 = Close File(refnum=w299, error in=w301) -> (error out=w300:errorcluster)  [unwired: 1 out]
      n145 = call <vilib>:"Simple Error Handler.vi"("error in (no error)"=w300) -> ()  [unwired: 4 in, 5 out]
    }
    frame Disabled {
    }
  }
  n146 = Build Path(base path=w1, name or relative path=w8) -> (appended path=w3:path)
  n147 = Build Array(w14, w13) -> (w2:string[][])
  n148 = call <instrlib>:"Close.vi"("error in (no error)"=w20, "Mercury Reference"=w19) -> ("error out"=→"error out":errorcluster)  [unwired: 9 in]
  n149 = call-poly <vilib>:"Write Delimited Spreadsheet.vi"("file path (dialog if empty)"=w3, "2D data"=w2, "append to file? (new file:F)"=TRUE, "transpose? (no:F)"=TRUE, "delimiter (\\t)"="" ("delimiter (\\t)")) -> ()  [unwired: 9 in, 2 out]
